vi "getUserEvents.vi"(11 "UserEvents in":refnum<class "UserEvents.lvclass">) -> (2 "UserEvents":T1, 3 "UserEvents out":refnum<class "UserEvents.lvclass">)   [LabVIEW 2016, in "UserEvents.lvclass"]
uses:
  UserEvents.lvclass
  Types/UserEvents.ctl
  Types/StateChangedEvent.ctl
  Types/Timestamp.ctl
  Types/SummaryStates.ctl
  Types/DetailedStates.ctl
  Types/ProcessCommandEvent.ctl
  Commands/Command/Command.lvclass
  Types/ShutdownEvent.ctl
  UserEvents.lvclass/UserEvents.ctl
  Types/M1M3SupportTypes.lvlib
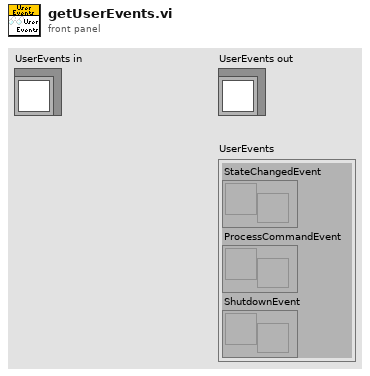
[diagram p1: front panel]
types:
  T1 = typedef "M1M3SupportTypes.lvlib/UserEvents.ctl" = cluster{"StateChangedEvent":refnum<user-event>, "ProcessCommandEvent":refnum<user-event>, "ShutdownEvent":refnum<user-event>}
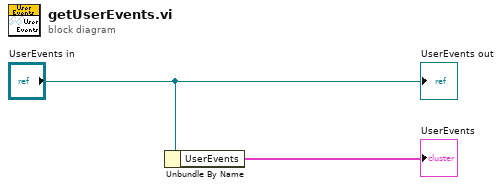
[diagram p0: block diagram]
diagram:
  n1 = Unbundle By Name("UserEvents in") -> ("UserEvents"=→"UserEvents":T1)
  "UserEvents out" <- "UserEvents in"
